vi "Main.vi"() -> ()   [LabVIEW 2021]
doc: "Please follow instructions on the right side of this VI.\nRequuieres: Lake Shore Cryotronics model 350 - to measure teperature on standard sensor and set temperature of testing space; SMU Keithley 2450 (2x) - for a four-wire measurements of a sensors rezistance."
uses:
  controls/Data.ctl
  controls/State.ctl
  <instrlib>/Lake Shore 350/Lake Shore 350.lvlib
  <instrlib>/Keithley 2450/Keithley 2450.lvlib
panel:
  in  "Ramp Rate (K/min)":dbl=10.0
  out "Last poit before (s)":dbl caption="Elapsed Time (s)"
  in  "Start imediatly":bool
  in  "Type":enum16{"Log", "Quadratic", "Cubic", "Linear"}(ring)
  in  "Number of points":i32=195
  out "Progress %":dbl(slide) caption="Horizontal Pointer Slide" scale=0.0..100.0
  out "Data":T1
  in  "Start point":dbl=302.0
  in  "End point":dbl=2.0
  in  "Two way calibration":bool
  in  "Use second SMUs":bool
  in  "Stop btn":bool
  in  "Start btn":bool
  in  "Instruments":T2={"TC"={"Port"="COM4", "Connected"=TRUE, "Ambient"=0.0, "VTI"=301.985, "Sample"=302.187, "Pot"=3.85785, "Trap"=41.8251, "VTI setpoint"=302.0, "VTI heater %"=0.0, "Last updated"=3726676112.779511}, "SMUs"=[{"Port"="USB0::0x05E6::0x2450::04408955::INSTR", "Sensor name"="X166279", "Connected"=FALSE, "Last updated"=3726676042.704634, "Value"=71.45189}, {"Port"="USB0::0x05E6::0x2450::04405250::INSTR", "Sensor name"="X137712", "Connected"=FALSE, "Last updated"=3726676066.0721498, "Value"=56.99837}]} {"SMUs"."Last updated" format="%<%H:%M:%S>T"; "TC"."Last updated" format="%<%H:%M:%S>T"}
  in  "End btn":bool
  out "Actual temperature chart":T3(graph)
  out "Rezistance graph":cluster{dbl[], dbl[]}[](graph)
  out "Message logs":string[](array[string])=["USB0::0x05E6::0x2450::04405250::INSTR connected.", "TC connected", "", "", "", "", "", "", "", "", "", "", "", "", "", "", "", "", "", ""]
  # "T=1,6*exp(0,0135*n)     where n is N in <1,"
  # "Guide:\n1. Before starting of program, setup instruments. Port, sensor name.\n2. Setup type of point distribution (linear for Pt sensors).\n3. setup start, end point, number of points (example: for cernox: cubic, 300 K, 2 K, 195)\nRecomend to set Start point to higher value than End point, but lower or equal to acutual value.\n4. Check use second SMU if you want to calibreate 2 sensors at once. \n5. When program is running, press START, to start measurement.\n6. Procedure takes few hours, datafile will be saved the in same directory from which program is run.\n7. When done, extrapolate curve by one point at each end (example: 310 K and 1.7 K; easy to do in Excel).\n8. Calculate logarithm with base 10 (Log10) for values of resitnace (column named as sensor name).\n9. Create a copy of older calibration file *.340, change name, open as text file, modify header, and replace values\nin column Units and Temperature (K) by calculated Log10 of resistance and Standard [K] respectively. (better txt\neditors allows to use ALT for vertical selection)"
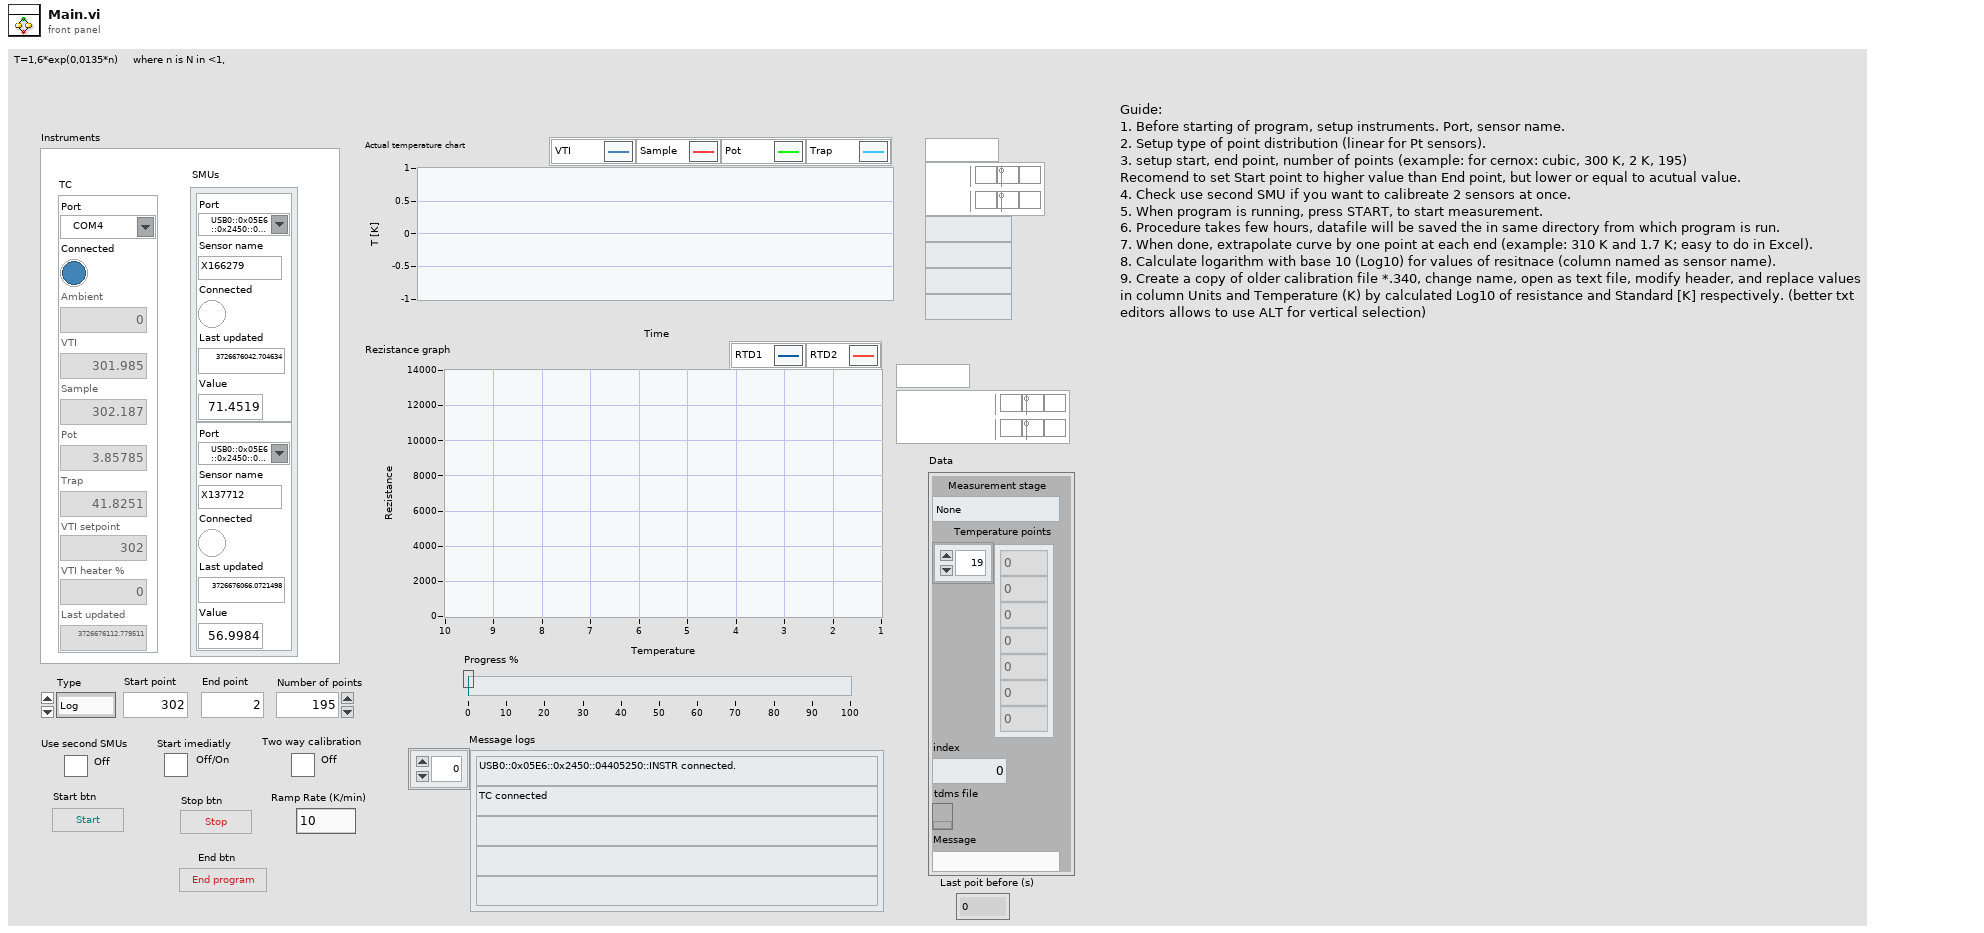
[diagram p1: front panel]
types:
  T1 = typedef "Data.ctl" = cluster{"Measurement stage":enum16{"None", "Wait to start", "Stage 1", "Interstage", "Stage 2", "Stopping"}, "Temperature points":dbl[], "index":i32, "tdms file":refnum<k34>, "Message":string}
  T2 = cluster{"TC":cluster{"Port":refnum<visa-resource-name>, "Connected":bool, "Ambient":dbl, "VTI":dbl, "Sample":dbl, "Pot":dbl, "Trap":dbl, "VTI setpoint":dbl, "VTI heater %":dbl, "Last updated":dbl}, "SMUs":cluster{"Port":refnum<visa-resource-name>, "Sensor name":string, "Connected":bool, "Last updated":dbl, "Value":dbl}[]}
  T3 = cluster{"VTI":dbl, "Sample":dbl, "Trap":dbl, "Pot":dbl}
  T4 = typedef "State.ctl" = enum16{"Initialize", "Connect to TC", "Disconnect TC", "Connect to SMU", "Disconnect SMU ", "Set TC", "Read TC", "Set SMU", "Read SMU", "Wait for Event", "Start measurement", "Save datapoint", "End measurement", "Stop program"}
  T5 = enum16{"None", "Wait to start", "Stage 1", "Interstage", "Stage 2", "Stopping"}
  T6 = cluster{"Baud Rate":u32, "Parity":u16, "Data Bits":u16, "Stop Bits":u16, "Flow Control":u16}
  T7 = cluster{"Port":refnum<visa-resource-name>, "Sensor name":string, "Connected":bool, "Last updated":dbl, "Value":dbl}[]
  T8 = cluster{"Port":refnum<visa-resource-name>, "Sensor name":string, "Connected":bool, "Last updated":dbl, "Value":dbl}
  T9 = cluster{"Port":refnum<visa-resource-name>, "Connected":bool, "Ambient":dbl, "VTI":dbl, "Sample":dbl, "Pot":dbl, "Trap":dbl, "VTI setpoint":dbl, "VTI heater %":dbl, "Last updated":dbl}
  T10 = cluster{"Port":refnum<visa-resource-name>, "Connected":bool, "Ambient":dbl, "VTI":dbl, "Sample":dbl, "Trap":dbl, "Pot":dbl, "VTI setpoint":dbl, "VTI heater %":dbl, "Last updated":dbl}
  T11 = cluster{"TC":cluster{"Port":refnum<visa-resource-name>, "Connected":bool, "Ambient":dbl, "VTI":dbl, "Sample":dbl, "Trap":dbl, "Pot":dbl, "VTI setpoint":dbl, "VTI heater %":dbl, "Last updated":dbl}, "SMUs":cluster{"Port":refnum<visa-resource-name>, "Sensor name":string, "Connected":bool, "Last updated":dbl, "Value":dbl}[]}
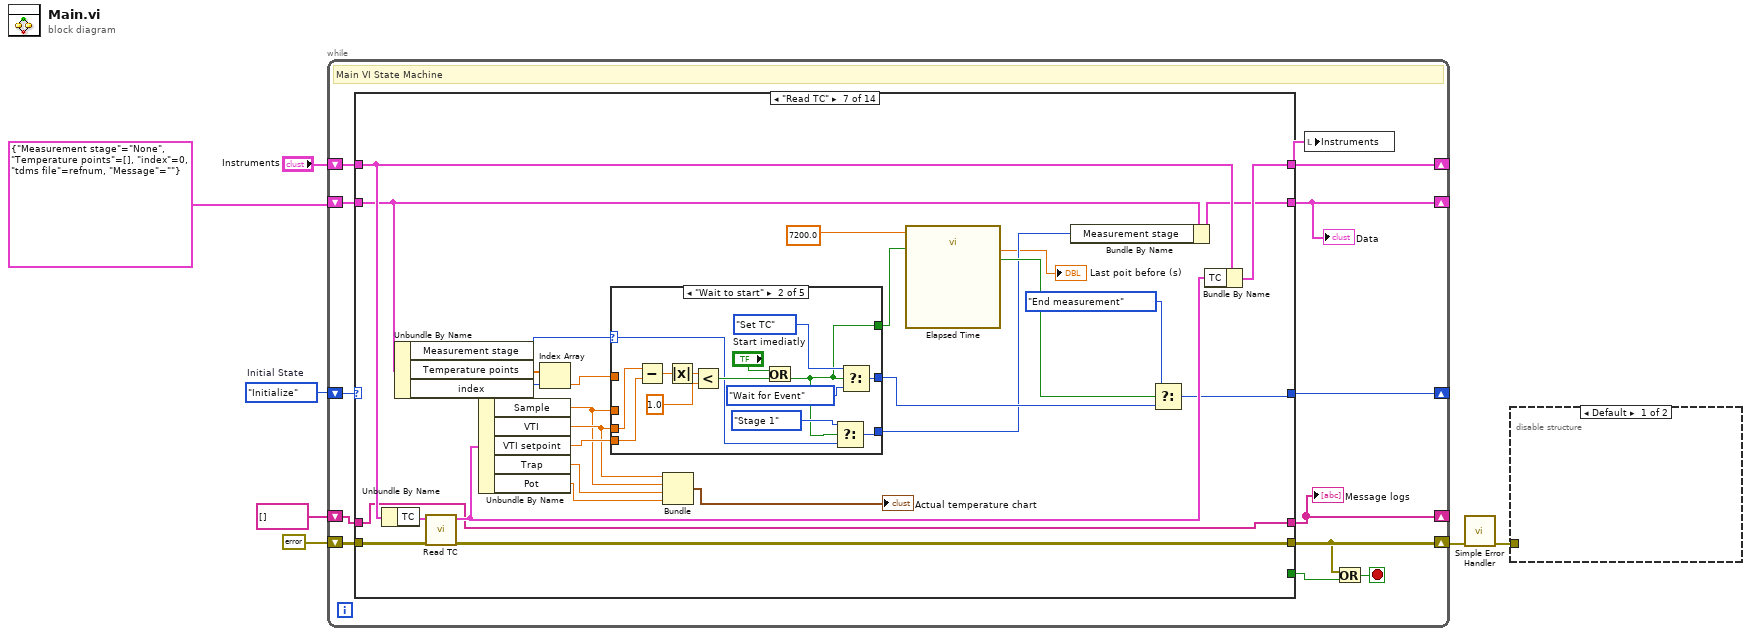
[diagram p0: block diagram]
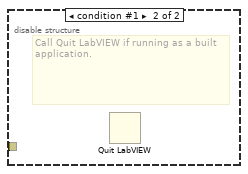
[diagram p2: hidden frame]
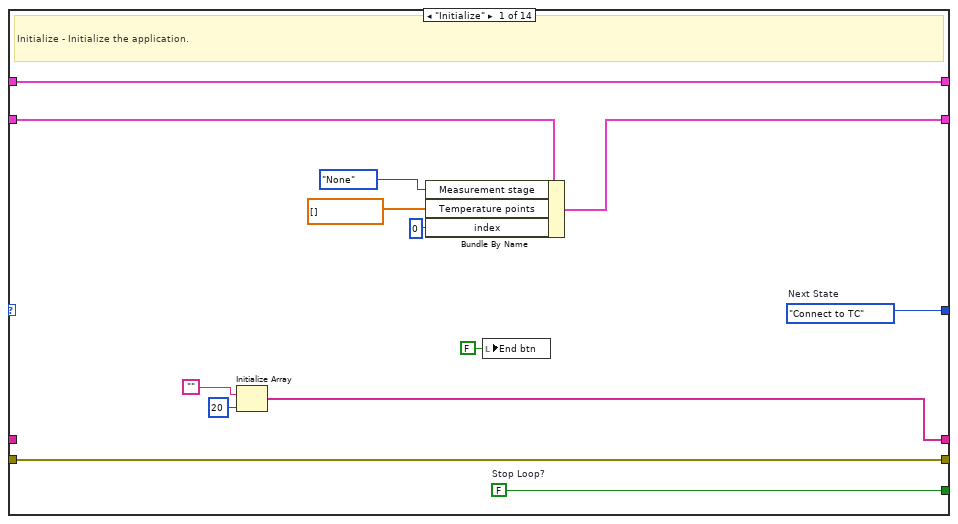
[diagram p3: hidden frame]
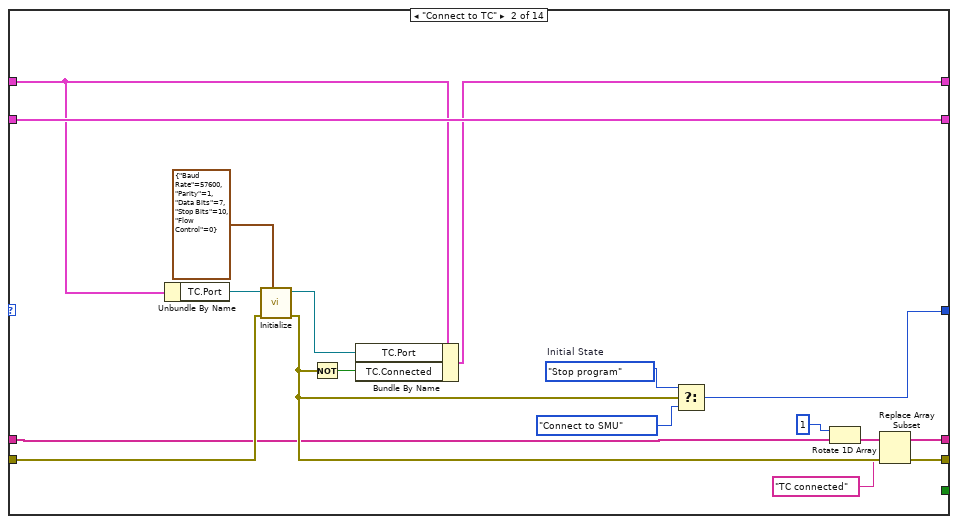
[diagram p4: hidden frame]
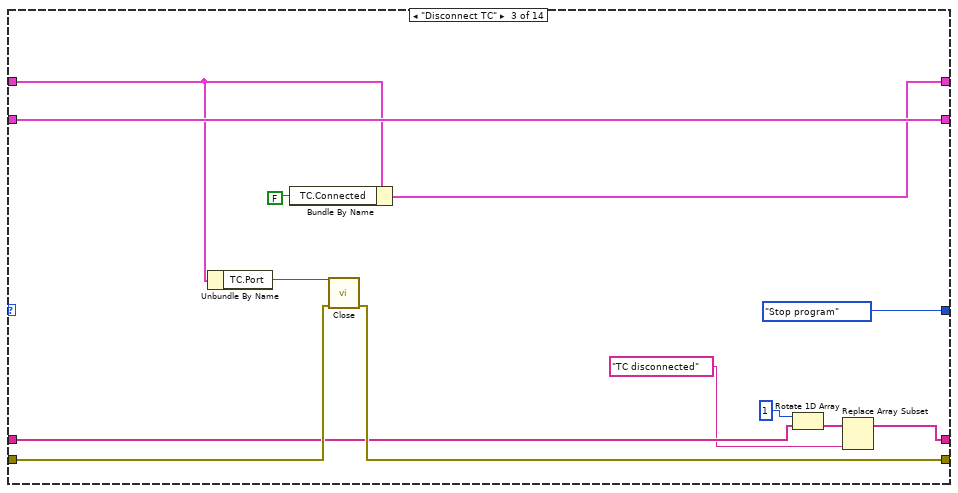
[diagram p5: hidden frame]
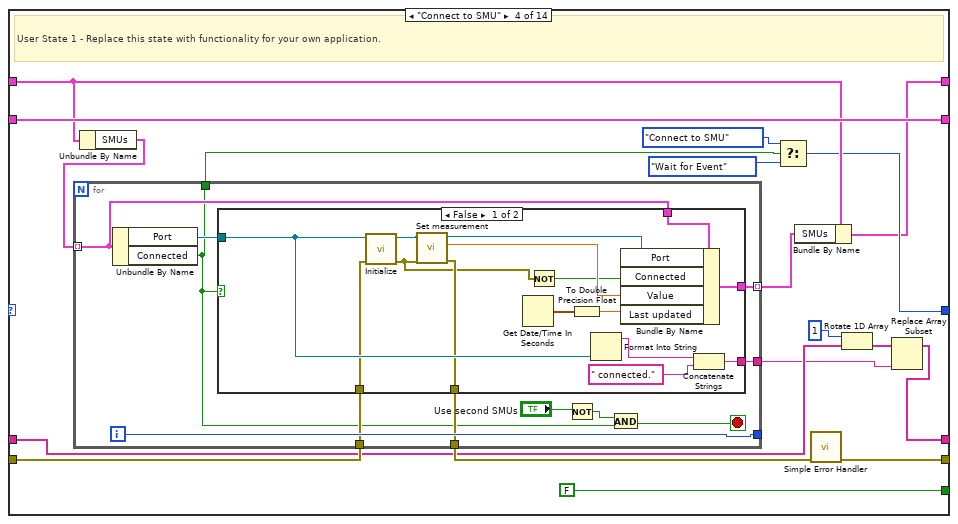
[diagram p6: hidden frame]
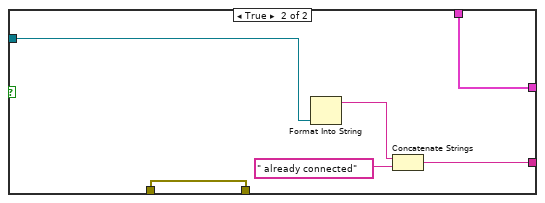
[diagram p7: hidden frame]
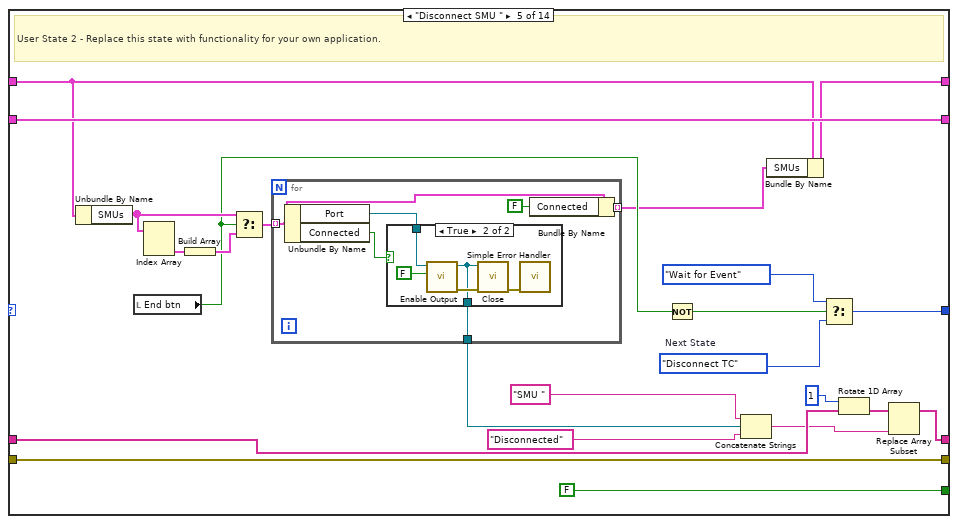
[diagram p8: hidden frame]
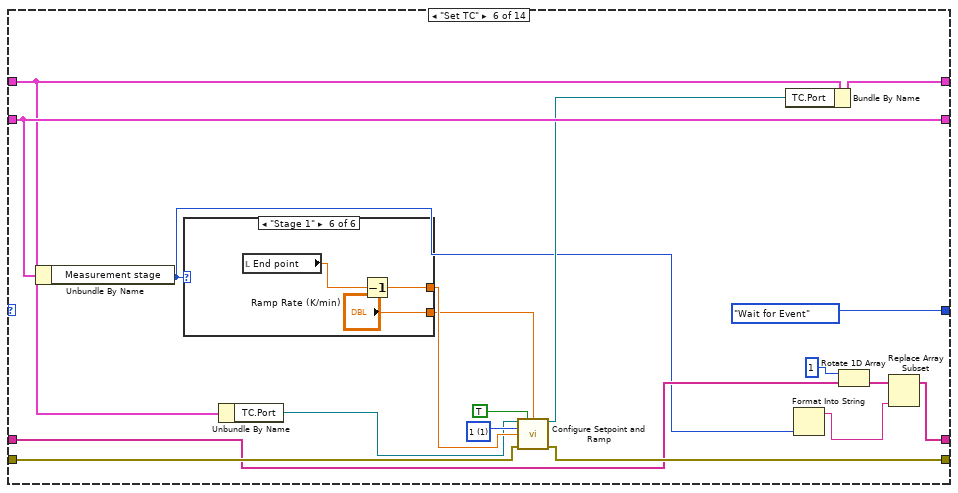
[diagram p10: hidden frame]
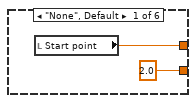
[diagram p11: hidden frame]
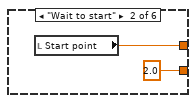
[diagram p12: hidden frame]
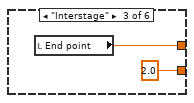
[diagram p13: hidden frame]
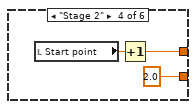
[diagram p14: hidden frame]
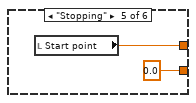
[diagram p15: hidden frame]
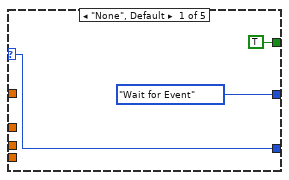
[diagram p16: hidden frame]
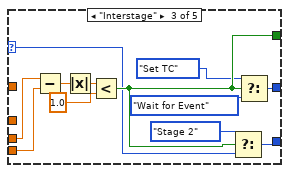
[diagram p17: hidden frame]
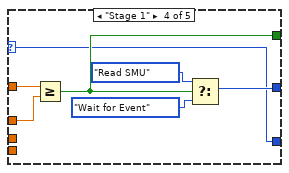
[diagram p18: hidden frame]
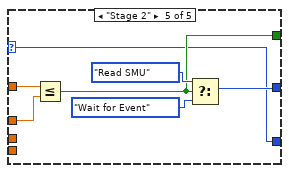
[diagram p19: hidden frame]
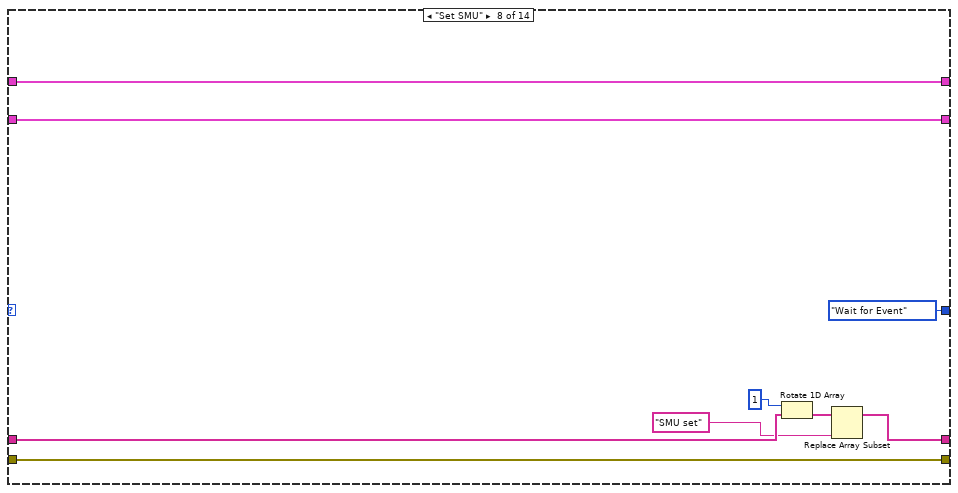
[diagram p20: hidden frame]
diagram:
  w7 = State."Initialize"  # Initial State
  n1 = while {
    shift-right: [w18] -> _
    shift-left: w7 -> [w19]
    shift-right: [w16] -> _
    shift-left: T1 {"Measurement stage"=enum."None", "Temperature points"=[], "index"=0, "tdms file"=refnum, "Message"=""} ("Data") -> [w17]
    shift-right: [w12] -> w4
    shift-left: errorcluster {"status"=FALSE, "code"=0, "source"=""} ("error constant") -> [w15]
    shift-right: [w10] -> _
    shift-left: "Instruments" -> [w11]
    shift-right: [w8] -> _
    shift-left: string[] [] -> [w9]
    stop <- w13 stop-if-true
    # "Main VI State Machine"
    n2 = case shown="\"Read TC\"" w19 {
      tunnel: [w32 w41 State."Stop program" ("(Value Not Used)") w74 w132 State."Wait for Event" ("(Value Not Used)") w191 State."Wait for Event" ("(Value Not Used)") State."Save datapoint" ("(Value Not Used)") w275 State."Set TC" ("(Value Not Used)") w341 w368 w390] -> w18
      tunnel: [w31 _ _ FALSE ("Stop Loop?") FALSE ("Stop Loop?") _ _ _ _ w274 _ _ _ w388] -> w14
      tunnel: w17 -> [w30 w49 w62 w79 w134 w158 w201 w258 w265 w273 w310 w343 w367 w389]
      tunnel: [w29 w49 w62 w79 w134 w158 w188 w258 w265 w272 w325 w335 w358 w389] -> w16
      tunnel: w15 -> [w28 w46 w61 w71 w133 w163 w205 w257 w260 w271 w314 w336 w352 w387]
      tunnel: [w28 w43 w59 w69 w133 w162 w206 w257 w264 w270 w313 w337 w353 w387] -> w12
      tunnel: [w27 w38 w56 w73 w114 w157 w202 w256 w263 w269 w324 w338 w369 w386] -> w10
      tunnel: w11 -> [w27 w45 w57 w78 w127 w149 w203 w256 w259 w269 w324 w338 w369 w386]
      tunnel: [w21 w34 w52 w64 w119 w151 w186 w252 w261 w267 w305 w328 w348 w383] -> w8
      tunnel: w9 -> [_ w37 w51 w66 w121 w153 w186 w251 w261 w267 w304 w329 w349 w385]
      frame "Initialize" {
        w31 = FALSE  # Stop Loop?
        w32 = State."Connect to TC"  # Next State
        # "Initialize - Initialize the application."
        n3 = Initialize Array("", 20 ("dimension size")) -> (w21:string[])
        n4 = Bundle By Name(cluster=w30, "Measurement stage"=T5."None", "Temperature points"=dbl[] [], "index"=0) -> (w29:T1)
        n5 = local write "End btn"(FALSE ("End btn")) -> ()
      }
      frame "Connect to TC" {
        w42 = State."Stop program"  # Initial State
        n6 = Unbundle By Name(w45) -> ("TC.Port"=w48:refnum<visa-resource-name>)
        n7 = call <instrlib>:"Initialize.vi"("Serial Configuration"=T6 {"Baud Rate"=57600, "Parity"=1, "Data Bits"=7, "Stop Bits"=10, "Flow Control"=0}, "error in (no error)"=w46, "VISA resource name"=w48) -> ("error out"=w43:errorcluster, "VISA resource name out"=w39:refnum<visa-resource-name>)  [unwired: 7 in]
        n8 = Not(x=w43) -> (.not. x?=w44:bool)
        n9 = Bundle By Name(cluster=w45, "TC.Port"=w39, "TC.Connected"=w44) -> (w38:T2)
        n10 = Select(t=w42, s=w43, f=State."Connect to SMU") -> (s? t:f=w41:T4)
        n11 = Rotate 1D Array(1:w37, 2:1 ("n")) -> (0:w36:string[])
        n12 = Replace Array Subset(array=w36, new element="TC connected") -> (w34:string[])  [unwired: 1 in]
      }
      frame "Disconnect TC" {
        n13 = Unbundle By Name(w57) -> ("TC.Port"=w60:refnum<visa-resource-name>)
        n14 = Bundle By Name(cluster=w57, "TC.Connected"=FALSE) -> (w56:T2)
        n15 = call <instrlib>:"Close.vi"("error in (no error)"=w61, "VISA resource name"=w60) -> ("error out"=w59:errorcluster)  [unwired: 9 in]
        n16 = Rotate 1D Array(1:w51, 2:1 ("n")) -> (0:w54:string[])
        n17 = Replace Array Subset(array=w54, new element="TC disconnected") -> (w52:string[])  [unwired: 1 in]
      }
      frame "Connect to SMU" {
        # "User State 1 - Replace this state with functionality for your own application."
        n18 = Unbundle By Name(w78) -> ("SMUs"=w77:T7)
        n19 = for {
          tunnel: w77 -> [w89] mode=indexing
          tunnel: [w90] -> _
          tunnel: [w88] -> w65
          tunnel: [w84] -> w72
          tunnel: w71 -> [w83]
          tunnel: [w82] -> w70 mode=indexing
          tunnel: [w81] -> w63
          i -> [w90]
          stop <- w87 stop-if-true
          n20 = Unbundle By Name(w89) -> ("Port"=w91:refnum<visa-resource-name>, "Connected"=w81:bool)
          n21 = case shown="False" w81 {
            tunnel: w91 -> [w99 w112]
            tunnel: w89 -> [w105 w107]
            tunnel: [w97 w109] -> w88
            tunnel: [w93 w108] -> w84
            tunnel: w83 -> [w96 w108]
            tunnel: [w95 w107] -> w82
            frame False {
              n22 = call <instrlib>:"Initialize.vi"("error in (no error)"=w96, "VISA resource name"=w99) -> ("error out"=w92:errorcluster, "VISA resource name out"=w106:refnum<visa-resource-name>)  [unwired: 8 in]
              n23 = call "Set measurement.vi"("error in (no error)"=w92, "VISA resource name"=w106) -> ("error out"=w93:errorcluster, "Value"=w101:dbl, "VISA resource name out"=w104:refnum<visa-resource-name>)  [unwired: 5 in, 2 out]
              n24 = Get Date/Time In Seconds() -> (seconds since 1Jan1904=w103:timestamp)
              n25 = Not(x=w92) -> (.not. x?=w94:bool)
              n26 = To Double Precision Float(number=w103) -> (double precision float=w102:dbl)
              n27 = Format Into String(w99) -> (resulting string=w100:string)  [unwired: 3 in, 1 out]
              n28 = Bundle By Name(cluster=w105, "Port"=w104, "Connected"=w94, "Value"=w101, "Last updated"=w102) -> (w95:T8)
              n29 = Concatenate Strings(w100, " connected.") -> (w97:string)
            }
            frame True {
              n30 = Format Into String(w112) -> (resulting string=w110:string)  [unwired: 3 in, 1 out]
              n31 = Concatenate Strings(w110, " already connected") -> (w109:string)
            }
          }
          n32 = Not(x="Use second SMUs") -> (.not. x?=w85:bool)
          n33 = And(x=w85, y=w81) -> (x .and. y?=w87:bool)
        }
        n34 = Select(t=State."Connect to SMU" ("(Value Not Used)"), s=w63, f=State."Wait for Event") -> (s? t:f=w74:T4)
        n35 = Bundle By Name(cluster=w78, "SMUs"=w70) -> (w73:T2)
        n36 = call <vilib>:"Simple Error Handler.vi"("error in (no error)"=w72) -> ("error out"=w69:errorcluster)  [unwired: 4 in, 4 out]
        n37 = Rotate 1D Array(1:w66, 2:1 ("n")) -> (0:w68:string[])
        n38 = Replace Array Subset(array=w68, new element=w65) -> (w64:string[])  [unwired: 1 in]
      }
      frame "Disconnect SMU " {
        w118 = State."Disconnect TC"  # Next State
        # "User State 2 - Replace this state with functionality for your own application."
        n39 = Unbundle By Name(w127) -> ("SMUs"=w125:T7)
        n40 = local read "End btn"() -> (w117:bool)
        n41 = Index Array(array=w125) -> (element #2=w115:T8)  [unwired: 2 in, 1 out]
        n42 = Build Array(w115) -> (w126:T7)
        n43 = Select(t=w125, s=w117, f=w126) -> (s? t:f=w124:T7)
        n44 = for {
          tunnel: [w141] -> w128
          tunnel: w124 -> [w138] mode=indexing
          tunnel: [w136] -> w113 mode=indexing
          n45 = Unbundle By Name(w138) -> ("Port"=w140:refnum<visa-resource-name>, "Connected"=w139:bool)
          n46 = case shown="True" w139 {
            tunnel: [w142 w145] -> w141
            tunnel: w140 -> [w142 w144]
            frame False {
            }
            frame True {
              n47 = call <instrlib>:"Enable Output.vi"("Enable Output (T: Enable)"=FALSE, "VISA resource name"=w144) -> ("error out"=w147:errorcluster, "VISA resource name out"=w145:refnum<visa-resource-name>)  [unwired: 8 in]
              n48 = call <instrlib>:"Close.vi"("error in (no error)"=w147, "VISA resource name"=w145) -> ("error out"=w143:errorcluster)  [unwired: 9 in]
              n49 = call <vilib>:"Simple Error Handler.vi"("error in (no error)"=w143) -> ()  [unwired: 4 in, 5 out]
            }
          }
          n50 = Bundle By Name(cluster=w138, "Connected"=FALSE) -> (w136:T8)
        }
        n51 = Not(x=w117) -> (.not. x?=w116:bool)
        n52 = Concatenate Strings("SMU ", w128, "Disconnected") -> (w120:string)
        n53 = Bundle By Name(cluster=w127, "SMUs"=w113) -> (w114:T2)
        n54 = Select(t=State."Wait for Event", s=w116, f=w118) -> (s? t:f=w132:T4)
        n55 = Rotate 1D Array(1:w121, 2:1 ("n")) -> (0:w123:string[])
        n56 = Replace Array Subset(array=w123, new element=w120) -> (w119:string[])  [unwired: 1 in]
      }
      frame "Set TC" {
        w165 = u16 1 items=["1"=1, "2"=2, "3"=3, "4"=4] ("Output's Control Loop (1:1)")
        n57 = Unbundle By Name(w158) -> ("Measurement stage"=w150:T5)
        n58 = case shown="\"Stage 1\"" w150 {
          tunnel: [w167 w169 w171 w173 w176 w178] -> w160
          tunnel: [2.0 ("Ramp Rate (0.0)") 2.0 ("Ramp Rate (0.0)") 2.0 ("Ramp Rate (0.0)") 2.0 ("Ramp Rate (0.0)") 0.0 ("Ramp Rate (0.0)") "Ramp Rate (K/min)"] -> w148
          frame "None", Default {
            n59 = local read "Start point"() -> (w167:dbl)
          }
          frame "Wait to start" {
            n60 = local read "Start point"() -> (w169:dbl)
          }
          frame "Interstage" {
            n61 = local read "End point"() -> (w171:dbl)
          }
          frame "Stage 2" {
            n62 = local read "Start point"() -> (w174:dbl)
            n63 = Increment(x=w174) -> (x+1=w173:dbl)
          }
          frame "Stopping" {
            n64 = local read "Start point"() -> (w176:dbl)
          }
          frame "Stage 1" {
            n65 = local read "End point"() -> (w179:dbl)
            n66 = Decrement(x=w179) -> (x-1=w178:dbl)
          }
        }
        n67 = Unbundle By Name(w149) -> ("TC.Port"=w159:refnum<visa-resource-name>)
        n68 = call <instrlib>:"Configure Setpoint and Ramp.vi"("VISA resource name"=w159, "Enable Setpoint Ramping  (F: Disable)"=TRUE, "Ramp Rate (0.0)"=w148, "Output's Control Loop (1:1)"=w165, "Setpoint (0.00000)"=w160, "error in (no error)"=w163) -> ("VISA resource name out"=w156:refnum<visa-resource-name>, "error out"=w162:errorcluster)  [unwired: 8 in]
        n69 = Bundle By Name(cluster=w149, "TC.Port"=w156) -> (w157:T2)
        n70 = Format Into String(w150) -> (resulting string=w152:string)  [unwired: 3 in, 1 out]
        n71 = Rotate 1D Array(1:w153, 2:1 ("n")) -> (0:w155:string[])
        n72 = Replace Array Subset(array=w155, new element=w152) -> (w151:string[])  [unwired: 1 in]
      }
      frame "Read TC" {
        n73 = Unbundle By Name(w203) -> ("TC"=w204:T9)
        n74 = Unbundle By Name(w201) -> ("Measurement stage"=w198:T5, "Temperature points"=w200:dbl[], "index"=w199:i32)
        n75 = call "Read TC.vi"("error in (no error)"=w205, "TC in"=w204) -> ("error out"=w206:errorcluster, "TC out"=w195:T10)  [unwired: 8 in]
        n76 = Unbundle By Name(w195) -> ("Sample"=w184:dbl, "VTI"=w185:dbl, "VTI setpoint"=w192:dbl, "Trap"=w182:dbl, "Pot"=w181:dbl)
        n77 = Index Array(array=w200, index=w199) -> (element=w196:dbl)
        n78 = case shown="\"Wait to start\"" w198 {
          selector: w198 -> [w207 w212 w224 w236 w243]
          tunnel: [State."Wait for Event" ("(Value Not Used)") w223 w235 w241 w248] -> w197
          tunnel: w196 -> [_ _ _ w239 w246]
          tunnel: w184 -> [_ _ _ w238 w245]
          tunnel: [TRUE w211 w229 w237 w244] -> w194
          tunnel: w185 -> [_ w219 w231 _ _]
          tunnel: w192 -> [_ w218 w230 _ _]
          tunnel: [w207 w216 w228 w236 w243] -> w187
          frame "None", Default {
          }
          frame "Wait to start" {
            n79 = Subtract(x=w219, y=w218) -> (x-y=w222:dbl)
            n80 = Absolute Value(x=w222) -> (abs(x)=w220:dbl)
            n81 = Less?(x=w220, y=1.0) -> (x < y?=w217:bool)
            n82 = Or(x="Start imediatly", y=w217) -> (x .or. y?=w211:bool)
            n83 = Select(t=T5."Stage 1" ("Measurement stage"), s=w211, f=w212) -> (s? t:f=w216:T5)
            n84 = Select(t=State."Set TC" ("f"), s=w211, f=State."Wait for Event") -> (s? t:f=w223:T4)
          }
          frame "Interstage" {
            n85 = Subtract(x=w231, y=w230) -> (x-y=w234:dbl)
            n86 = Absolute Value(x=w234) -> (abs(x)=w232:dbl)
            n87 = Less?(x=w232, y=1.0) -> (x < y?=w229:bool)
            n88 = Select(t=T5."Stage 2" ("Measurement stage"), s=w229, f=w224) -> (s? t:f=w228:T5)
            n89 = Select(t=State."Set TC" ("f"), s=w229, f=State."Wait for Event") -> (s? t:f=w235:T4)
          }
          frame "Stage 1" {
            n90 = Greater Or Equal?(x=w239, y=w238) -> (x >= y?=w237:bool)
            n91 = Select(t=State."Read SMU", s=w237, f=State."Wait for Event") -> (s? t:f=w241:T4)
          }
          frame "Stage 2" {
            n92 = Less Or Equal?(x=w246, y=w245) -> (x <= y?=w244:bool)
            n93 = Select(t=State."Read SMU", s=w244, f=State."Wait for Event") -> (s? t:f=w248:T4)
          }
        }
        n94 = Bundle("VTI"=w185, "Sample"=w184, "Trap"=w182, "Pot"=w181) -> (→"Actual temperature chart":T3)  [unwired: 1 in]
        n95 = call "Elapsed Time"("Time Target (s)"=7200.0, "Reset"=w194) -> ("Elapsed Time (s)"=→"Last poit before (s)":dbl, "Time has Elapsed"=w190:bool)  [unwired: 10 in, 6 out]
        n96 = Bundle By Name(cluster=w201, "Measurement stage"=w187) -> (w188:T1)
        n97 = Select(t=State."End measurement", s=w190, f=w197) -> (s? t:f=w191:T4)
        n98 = Bundle By Name(cluster=w203, "TC"=w195) -> (w202:T2)
      }
      frame "Set SMU" {
        n99 = Rotate 1D Array(1:w251, 2:1 ("n")) -> (0:w254:string[])
        n100 = Replace Array Subset(array=w254, new element="SMU set" ("new element/subarray")) -> (w252:string[])  [unwired: 1 in]
      }
      frame "Read SMU" {
        n101 = local read "Use second SMUs"() -> (w266:bool)
        n102 = call "Read SMU.vi"("error in (no error)"=w260, "Instruments in"=w259, "Use second SMUs"=w266) -> ("error out"=w264:errorcluster, "Instruments out"=w263:T11)  [unwired: 7 in]
      }
      frame "Wait for Event" {
        w274 = FALSE  # Stop Loop?
        # "Wait for Event - Use an Event Structure to monitor the user interface for events that run different states of the state machine."
        n103 = event shown="[0] Timeout" {
          selector: _ -> [_ _ _ _ _ _]
          dyn-events: _ -> [_ _ _ _ _ _]
          timeout: 2000 -> [_ _ _ _ _ _]
          tunnel: [State."Read TC" ("Next State") w279 w289 w294 State."End measurement" ("Next State") w300] -> w275
          tunnel: w273 -> [w276 w284 w288 w293 w297 w299]
          tunnel: [w276 w284 w287 w292 w297 w299] -> w272
          tunnel: w271 -> [w278 w283 w285 w290 w296 w298]
          tunnel: [w278 w283 w285 w290 w296 w298] -> w270
          event Timeout {
            n104 = event-data() -> ()  [unwired: 1 in, 1 out]
          }
          event "Use second SMUs": Value Change {
            n105 = event-data() -> ("NewVal"=w280:bool)  [unwired: 1 in, 1 out]
            n106 = Select(t=State."Connect to SMU" ("Next State"), s=w280, f=State."Disconnect SMU " ("Next State")) -> (s? t:f=w279:T4)
          }
          event "Start point": Value Change {
            w289 = State."Set TC"  # Next State
            n107 = event-data() -> ()  [unwired: 1 in, 1 out]
            n108 = Bundle By Name(cluster=w288, "Message"="Running User State 1" ("Running User State 1")) -> (w287:T1)
          }
          event "Start btn": Value Change {
            w294 = State."Start measurement"  # Next State
            n109 = event-data() -> ()  [unwired: 1 in, 1 out]
            n110 = Bundle By Name(cluster=w293, "Message"="Running User State 2" ("Running User State 2")) -> (w292:T1)
          }
          event "Stop btn": Value Change {
            n111 = event-data() -> ()  [unwired: 1 in, 1 out]
          }
          event "End btn": Value Change {
            w300 = State."Disconnect SMU "  # Next State
            n112 = event-data() -> ()  [unwired: 1 in, 1 out]
          }
        }
      }
      frame "Start measurement" {
        n113 = Unbundle By Name(w324) -> ("SMUs"=w323:T7, "TC.Ambient"=w315:dbl)
        n114 = Index Array(array=w323) -> (element #1=w322:T8, element #2=w321:T8)  [unwired: 2 in]
        n115 = call "Generate tmp points.vi"("Type"="Type", "Number of points"="Number of points", "End point"="End point", "Start point"="Start point") -> ("Array"=w316:dbl[])  [unwired: 7 in]
        n116 = Unbundle By Name(w322) -> ("Sensor name"=w320:string)
        n117 = Unbundle By Name(w321) -> ("Sensor name"=w319:string)
        n118 = call "Create meas file with date.vi"("Start point"="Start point", "Ambient T"=w315, "End point"="End point", "error in (no error)"=w314, "Temperature setpoints"=w316, "Sensor 2 name"=w319, "Sensor 1 name"=w320) -> ("error out"=w313:errorcluster, "tdms file out"=w312:refnum<k34>)  [unwired: 3 in]
        n119 = local write "Rezistance graph"(cluster{dbl[], dbl[]}[] [] ("Rezistance graph")) -> ()
        n120 = invoke on="Actual temperature chart" class="WFChart (strict)" method="Reinit To Default"() -> ()  [unwired: 3 in, 3 out]
        n121 = Bundle By Name(cluster=w310, "Temperature points"=w316, "tdms file"=w312, "Measurement stage"=T5."Wait to start") -> (w325:T1)
        n122 = Rotate 1D Array(1:w304, 2:1 ("n")) -> (0:w307:string[])
        n123 = Replace Array Subset(array=w307, new element="Preparing to start measurement.") -> (w305:string[])  [unwired: 1 in]
      }
      frame "Save datapoint" {
        n124 = local read "Use second SMUs"() -> (w326:bool)
        n125 = local read "Rezistance graph"() -> (w333:cluster{dbl[], dbl[]}[])
        n126 = call "Save datapoint.vi"("Use second SMUs"=w326, "error in (no error)"=w336, "Data in"=w343, "Instruments"=w338, "graph data in"=w333) -> ("error out"=w337:errorcluster, "Is complete"=w339:bool, "Data out"=w335:T1, "Progress %"=→"Progress %":dbl, "Graph data out"=→"Rezistance graph":cluster{"Array":dbl[], "Array":dbl[]}[])  [unwired: 2 in]
        n127 = Rotate 1D Array(1:w329, 2:1 ("n")) -> (0:w331:string[])
        n128 = Select(t=State."End measurement" ("(Value Not Used)"), s=w339, f=State."Wait for Event") -> (s? t:f=w341:T4)
        n129 = Replace Array Subset(array=w331, new element="data point saved") -> (w328:string[])  [unwired: 1 in]
      }
      frame "End measurement" {
        n130 = Unbundle By Name(w367) -> ("Measurement stage"=w346:T5, "Temperature points"=w359:dbl[], "tdms file"=w362:refnum<k34>)  [unwired: 1 out]
        n131 = Format Into String(w346) -> (resulting string=w344:string)  [unwired: 3 in, 1 out]
        n132 = Concatenate Strings(w344, " finished") -> (w345:string)
        n133 = Equal?(x=w346, y=T5."Stage 1") -> (x = y?=w365:bool)
        n134 = TDMS Close(8:w352, 11:w362) -> (0:w360:errorcluster, 3:w361:path)
        n135 = And(x=w365, y="Two way calibration") -> (x .and. y?=w363:bool)
        n136 = case shown="False" w363 {
          tunnel: [State."Wait for Event" ("(Value Not Used)") State."Set TC" ("(Value Not Used)")] -> w368
          tunnel: w361 -> [_ w379]
          tunnel: w360 -> [w372 w378]
          tunnel: w359 -> [_ w377]
          tunnel: [T5."None" ("y") T5."Interstage" ("y")] -> w357
          tunnel: [_ w375] -> w356
          tunnel: [_ w374] -> w354
          tunnel: [w372 w373] -> w353
          frame False {
          }
          frame True {
            n137 = Reverse 1D Array(array=w377) -> (reversed array=w375:dbl[])
            n138 = TDMS Open(8:w378, 11:w379) -> (0:w373:errorcluster, 3:w374:refnum<k34>)  [unwired: 5 in]
          }
        }
        n139 = Bundle By Name(cluster=w367, "Measurement stage"=w357, "Temperature points"=w356, "index"=0, "tdms file"=w354) -> (w358:T1)
        n140 = Rotate 1D Array(1:w349, 2:1 ("n")) -> (0:w351:string[])
        n141 = Replace Array Subset(array=w351, new element=w345) -> (w348:string[])  [unwired: 1 in]
      }
      frame "Stop program" {
        w388 = TRUE  # Stop Loop?
        w390 = State."Stop program"  # (Value Not Used)
        # "#CodeNeeded - Add any required cleanup code here."
        # "The state value is not used here since this is the last iteration of the state machine loop."
        # "Exit - Exit the application."
        n142 = Rotate 1D Array(1:w385, 2:1 ("n")) -> (0:w384:string[])
        n143 = Replace Array Subset(array=w384, new element="Program stopped") -> (w383:string[])  [unwired: 1 in]
      }
    }
    "Message logs" <- w8
    "Data" <- w16
    n144 = local write "Instruments"(w10) -> ()
    n145 = Or(x=w12, y=w14) -> (x .or. y?=w13:bool)
  }
  n146 = call <vilib>:"Simple Error Handler.vi"("error in (no error)"=w4) -> ("error out"=w3:errorcluster)  [unwired: 4 in, 4 out]
  n147 = disable-structure shown="Default" {
    disable-tunnel: w3 -> [_ _]
    frame condition #0 (active) {
    }
    frame condition #1 {
      # "Call Quit LabVIEW if running as a built application."
      n148 = Quit LabVIEW() -> ()  [unwired: 1 in]
    }
  }
